vi "variables locales.vi"() -> ()   [LabVIEW 2020]
panel:
  out "initialized array":dbl[](array[numeric])
  out "String":string
  in  "stop":bool
  in  "Tank":dbl(slide) scale=0.0..10.0
  out "Foco1":bool
  in  "Pulsador1":bool
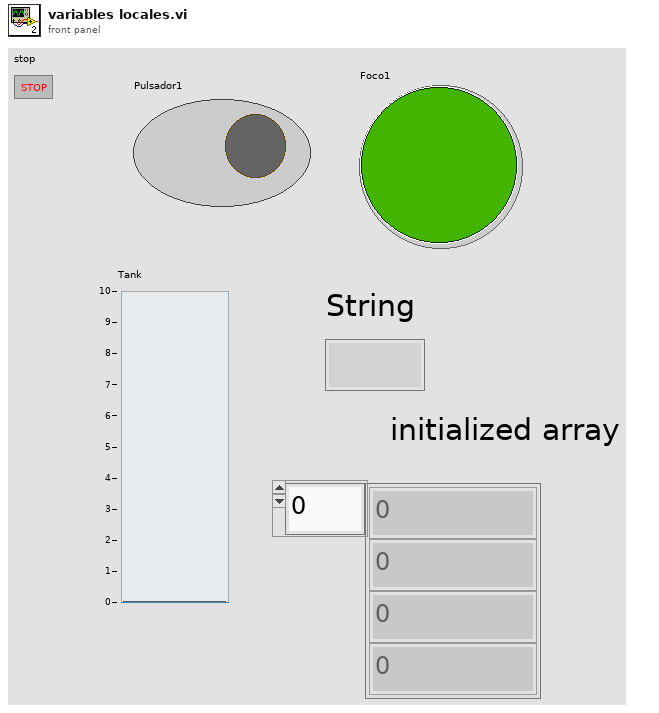
[diagram p1: front panel]
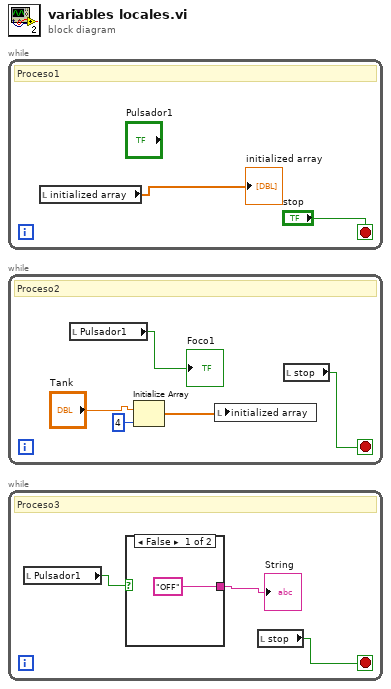
[diagram p0: block diagram]
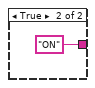
[diagram p2: hidden frame]
diagram:
  n1 = while {
    stop <- "stop" stop-if-true
    # "Proceso1"
    n2 = local read "initialized array"() -> (→"initialized array":dbl[])
  }
  n3 = while {
    stop <- w7 stop-if-true
    # "Proceso2"
    n4 = local read "Pulsador1"() -> (→"Foco1":bool)
    n5 = Initialize Array("Tank", 4 ("dimension size")) -> (w3:dbl[])
    n6 = local write "initialized array"(w3) -> ()
    n7 = local read "stop"() -> (w7:bool)
  }
  n8 = while {
    stop <- w10 stop-if-true
    # "Proceso3"
    n9 = local read "Pulsador1"() -> (w9:bool)
    n10 = case shown="False" w9 {
      tunnel: ["OFF" "ON"] -> w8
      frame False {
      }
      frame True {
      }
    }
    "String" <- w8
    n11 = local read "stop"() -> (w10:bool)
  }
